vi "examplePulseGeneration.vi"() -> ()   [LabVIEW 2023]
uses:
  <vilib>/measure/mamon.llb/Waveform Peak Detection for 1 Chan.vi
  <vilib>/measure/NI_MABase.lvlib
  <vilib>/measure/NI_MAPro.lvlib
panel:
  out "Locations":dbl[](array[numeric]) format="%.2p"
  out "Waveform Graph":waveform(dbl)(graph)
  out "# found":i32
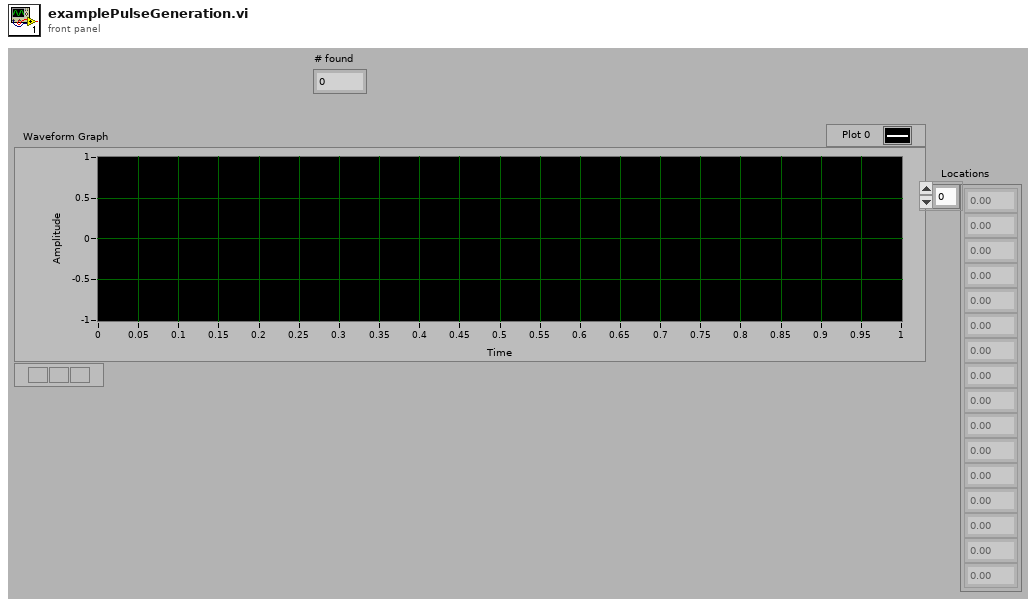
[diagram p1: front panel]
types:
  T1 = enum16{"Sine Wave", "Triangle Wave", "Square Wave", "Sawtooth Wave"}
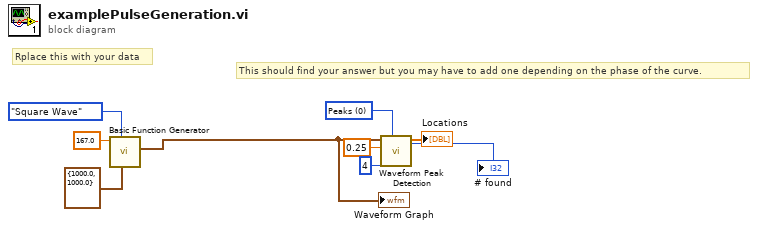
[diagram p0: block diagram]
diagram:
  w3 = u16 0 items=["Peaks", "Valleys"] ("peaks/valleys")
  # "This should find your answer but you may have to add one depending on the phase of the curve."
  # "Rplace this with your data"
  n1 = call <vilib>:"Basic Function Generator.vi"("sampling info"=cluster{"Fs":dbl, "#s":dbl} {"Fs"=1000.0, "#s"=1000.0}, "signal type"=T1."Square Wave", "frequency"=167.0) -> ("signal out"=w5:waveform(dbl))  [unwired: 6 in, 2 out]
  "Waveform Graph" <- w5
  n2 = call-poly <vilib>:"Waveform Peak Detection.vi"("peaks/valleys"=w3, "width"=4, "threshold"=0.25, "Signal In"=w5) -> ("Locations"=→"Locations":dbl[], "# found"=→"# found":i32)  [unwired: 3 in, 3 out]
